vi "Eth Status Write Starts.vi"(7 "Status Reference":T1, 8 "error in (no error)":errorcluster, 10 "Start":bool[](array[boolean]), 11 "Index":i32) -> (0 "error out":errorcluster)   [LabVIEW 2019, in "Eth Status.lvlib"]
uses:
  Eth Status.lvlib
  Ctl/Status.ctl
  MB_TCP2/MB_TCP_State.ctl
  MB_TCP2/MB_TCP.lvclass
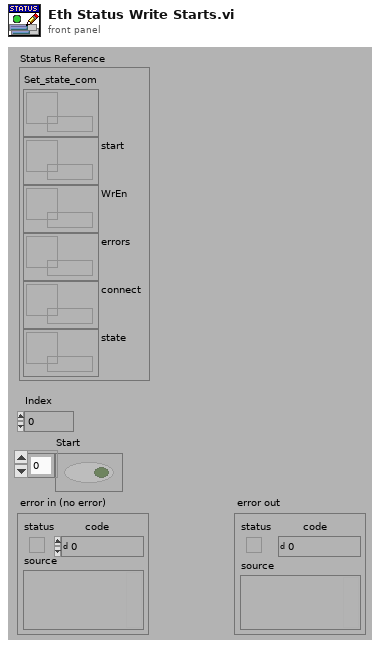
[diagram p1: front panel]
types:
  T1 = typedef "Eth Status.lvlib/Status.ctl" = cluster{"Set_state_com":refnum<data-value>, "start":refnum<data-value>, "WrEn":refnum<data-value>, "errors":refnum<data-value>, "connect":refnum<data-value>, "state":refnum<data-value>}
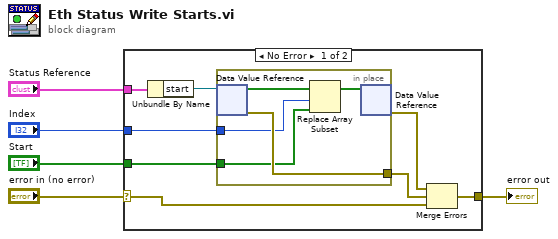
[diagram p0: block diagram]
diagram:
  n1 = case shown="No Error" "error in (no error)" {
    selector: "error in (no error)" -> [w6 w19]
    tunnel: [w11 w19] -> w4
    tunnel: "Index" -> [w13 _]
    tunnel: "Status Reference" -> [w12 _]
    tunnel: "Start" -> [w10 _]
    frame No Error {
      n2 = Unbundle By Name(w12) -> ("start"=w7:refnum<data-value>)
      n3 = in-place {
        in-place-border: w13 -> [w14]
        in-place-border: [w18] -> w9
        in-place-border: w10 -> [w15]
        n4 = in-place-dvr #1(w7) -> (w17:bool[], w18:errorcluster)
        n5 = Replace Array Subset(array=w17, new element=w15, index=w14) -> (w16:bool[])
        n6 = in-place-dvr #1(w16) -> (w8:errorcluster)  [unwired: 1 out]
      }
      n7 = Merge Errors(w8, w9, w6) -> (w11:errorcluster)
    }
    frame Error {
    }
  }
  "error out" <- w4
